vi "Unit Test FGV Spectrometer.vi"() -> ()   [LabVIEW 2013]
doc: "Use this template to build a producer/consumer design pattern with events to produce queue items. Use this design pattern instead of the User Interface Event Handler pattern for user interfaces when you want to execute code asynchronously in response to an event without slowing the user interface responsiveness."
uses:
  FGV Spectro Data.ctl
  Action Spectro.ctl
panel:
  in  "Set Device":bool
  out "Integration Time":dbl
  in  "Get Integration":bool
  in  "Device Set":i32
  out "Data out":T1
  out "Serial Number":string[](array[string])
  in  "Initialize":bool
  in  "Set Integ":dbl
  in  "Set Integration":bool
  in  "Get Spectre":bool
  in  "Disconnect":bool
  in  "Set Averange":bool
  in  "Averange":dbl
  in  "error in (no error)":errorcluster
  in  "Get WaveLength":bool
  out "error out":errorcluster
  in  "Connect":bool
  in  "stop":bool
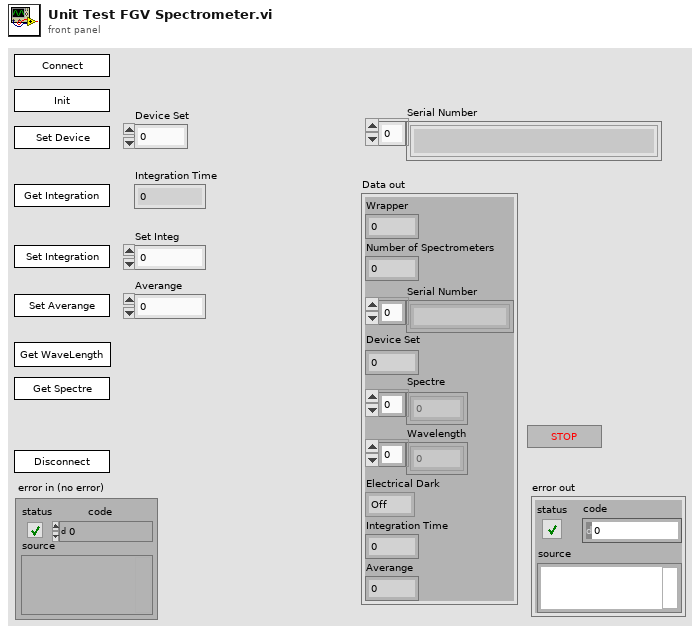
[diagram p1: front panel]
types:
  T1 = typedef "FGV Spectro Data.ctl" = cluster{"Wrapper":u32, "Number of Spectrometers":i32, "Serial Number":string[], "Device Set":i32, "Spectre":dbl[], "Wavelength":dbl[], "Electrical Dark":enum16{"Off", "On"}, "Integration Time":i32, "Averange":i32}
  T2 = typedef "Action Spectro.ctl" = enum16{"Connect", "Initialisation", "Set Device", "Set Intégration time", "Get integration Time", "Disable Noise Suppress", "Enable Noise Suppress", "Set Averange", "Get Spectrum", "Get WaveLength", "Abort", "Disconnect"}
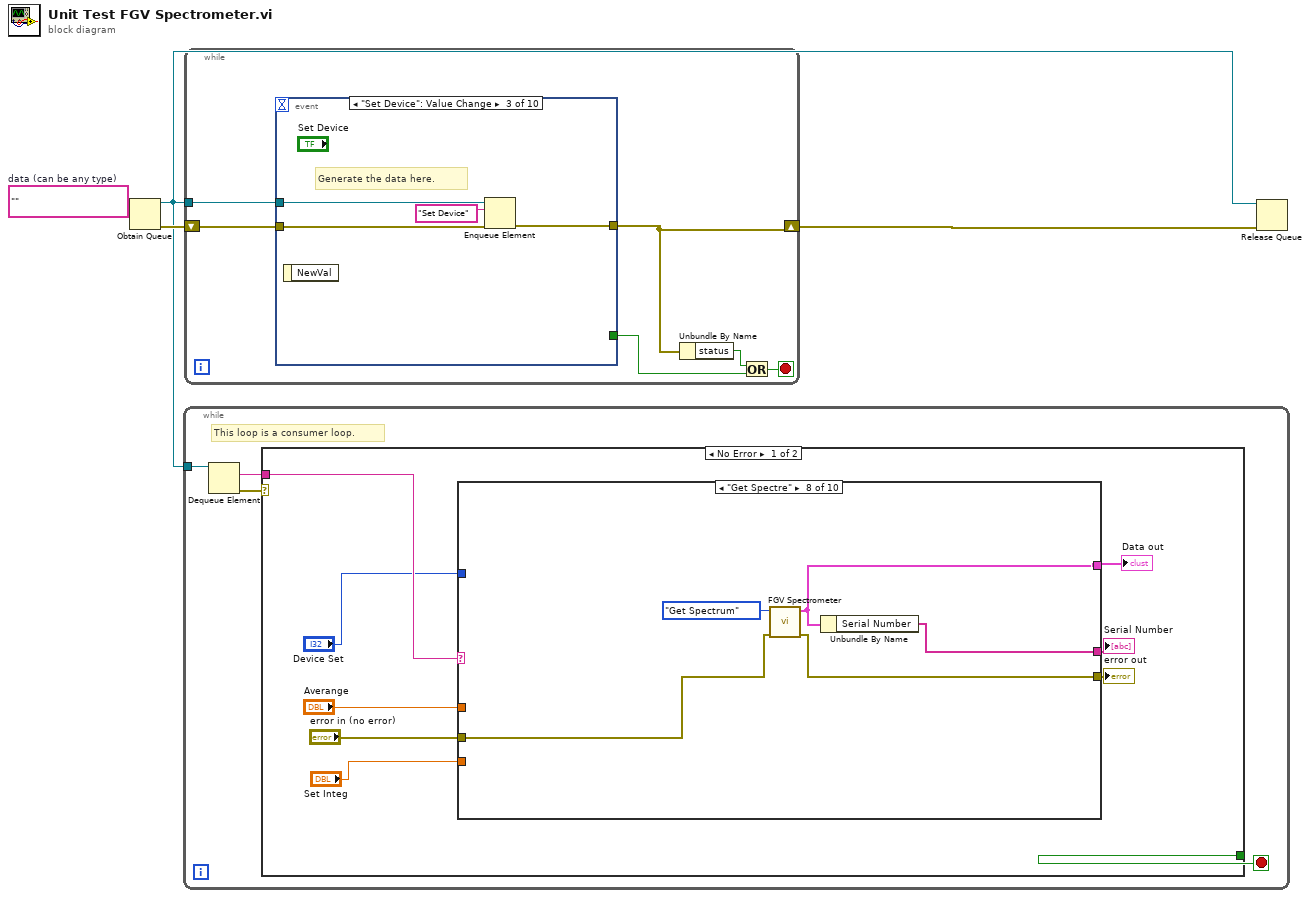
[diagram p0: block diagram]
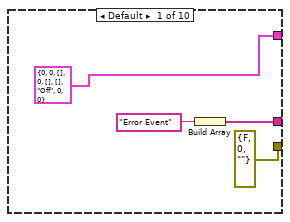
[diagram p2: hidden frame]
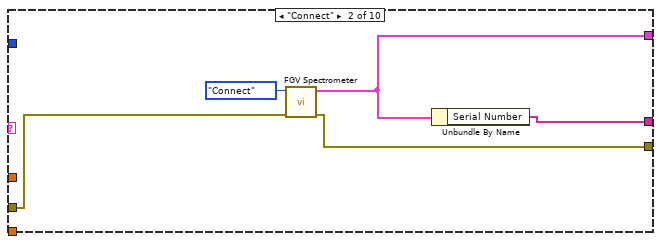
[diagram p3: hidden frame]
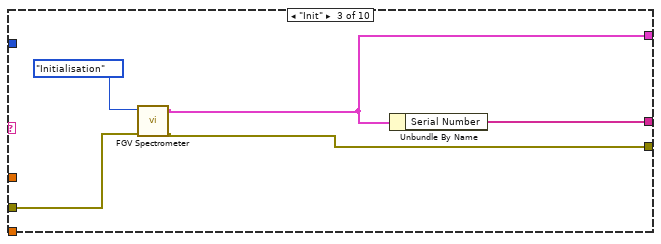
[diagram p4: hidden frame]
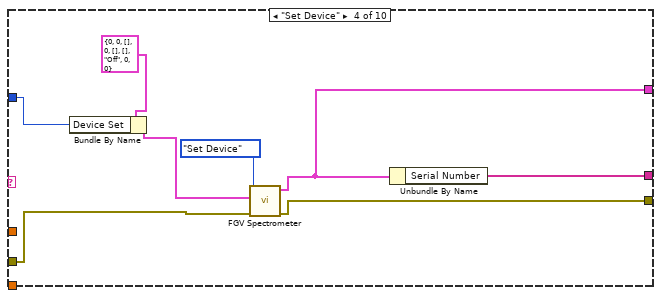
[diagram p5: hidden frame]
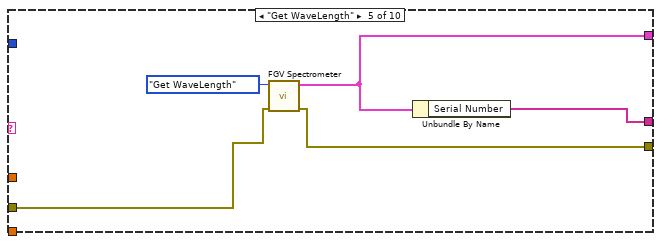
[diagram p6: hidden frame]
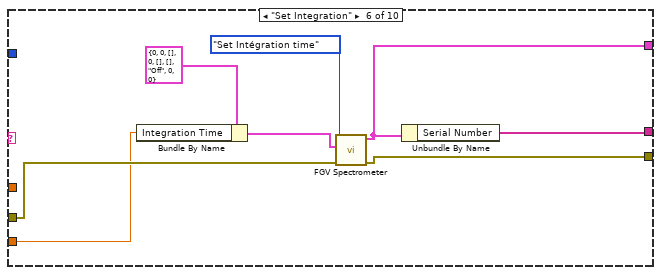
[diagram p7: hidden frame]
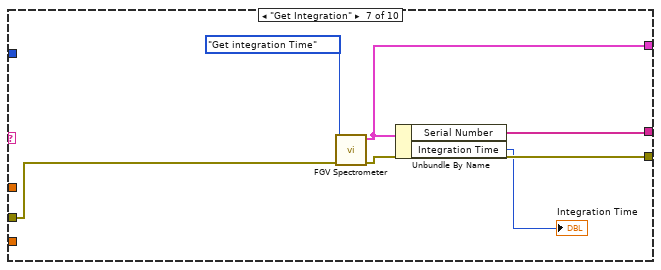
[diagram p8: hidden frame]
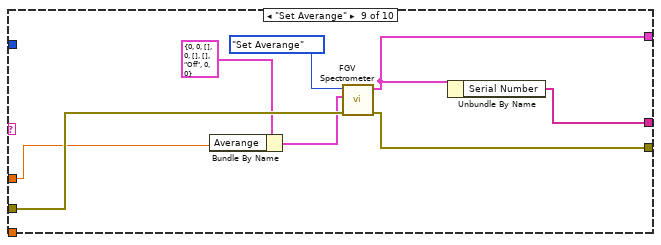
[diagram p9: hidden frame]
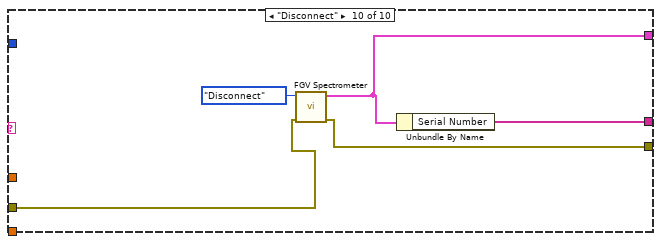
[diagram p10: hidden frame]
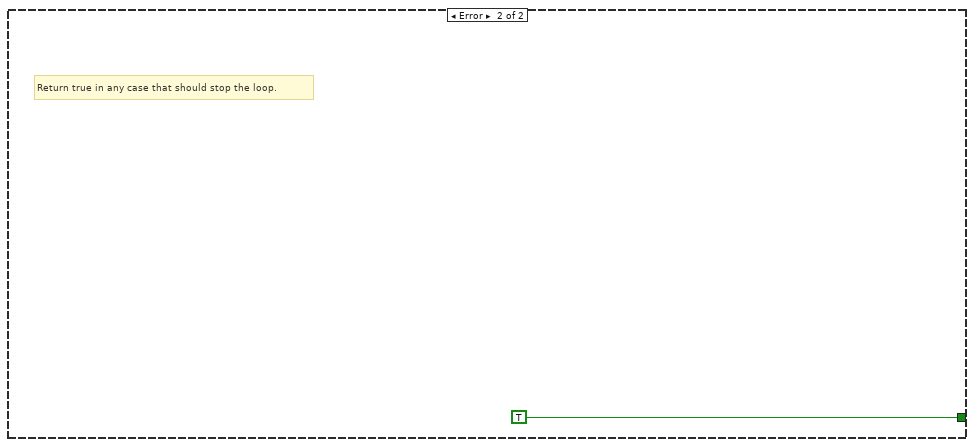
[diagram p11: hidden frame]
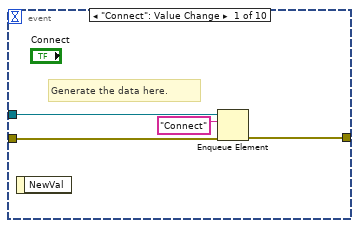
[diagram p12: hidden frame]
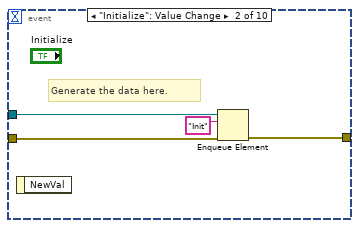
[diagram p13: hidden frame]
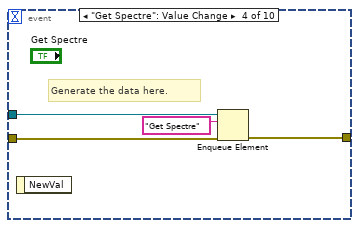
[diagram p14: hidden frame]
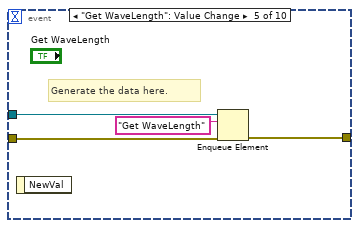
[diagram p15: hidden frame]
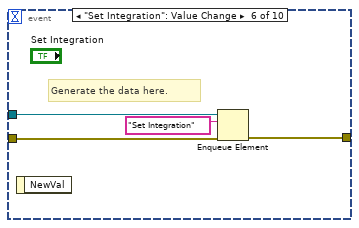
[diagram p16: hidden frame]
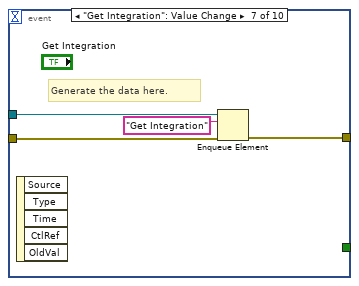
[diagram p17: hidden frame]
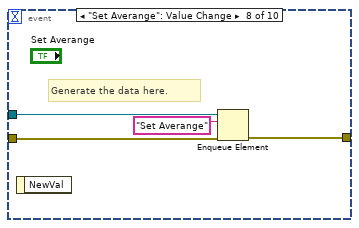
[diagram p18: hidden frame]
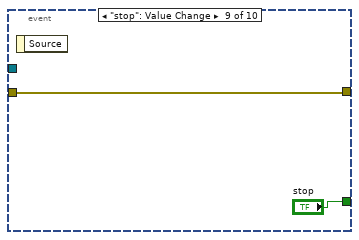
[diagram p19: hidden frame]
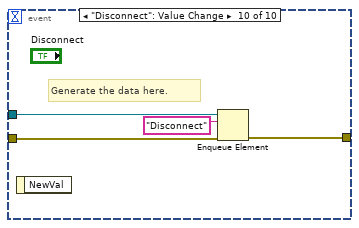
[diagram p20: hidden frame]
diagram:
  w2 = ""  # data (can be any type)
  n1 = Obtain Queue(element data type=w2) -> (queue out=w1:refnum<queue>, error out=w4:errorcluster)  [unwired: 4 in, 1 out]
  n2 = while {
    tunnel: w1 -> [w8]
    stop <- w5 stop-if-true
    # "This loop is a consumer loop."
    n3 = Dequeue Element(queue=w8) -> (element=w6:string, error out=w7:errorcluster)  [unwired: 2 in, 2 out]
    n4 = case shown="No Error" w7 {
      tunnel: w6 -> [w16 _]
      tunnel: [_ TRUE] -> w5
      frame No Error {
        n5 = case shown="\"Get Spectre\"" w16 {
          tunnel: [w17 w24 w29 w31 w41 w50 w56 w59 w67 w73] -> w11
          tunnel: [errorcluster {"status"=FALSE, "code"=0, "source"=""} ("error out") w23 w27 w32 w42 w49 w55 w61 w69 w74] -> w12
          tunnel: "error in (no error)" -> [_ w22 w30 w36 w43 w48 w54 w62 w70 w75]
          tunnel: "Averange" -> [_ _ _ _ _ _ _ _ w64 _]
          tunnel: "Set Integ" -> [_ _ _ _ _ w44 _ _ _ _]
          tunnel: [T1 {"Wrapper"=0, "Number of Spectrometers"=0, "Serial Number"=[], "Device Set"=0, "Spectre"=[], "Wavelength"=[], "Electrical Dark"=enum."Off", "Integration Time"=0, "Averange"=0} ("Data out") w21 w26 w33 w39 w51 w57 w60 w68 w72] -> w10
          tunnel: "Device Set" -> [_ _ _ w35 _ _ _ _ _ _]
          frame Default {
            n6 = Build Array("Error Event" ("Status")) -> (w17:string[])
          }
          frame "Connect" {
            n7 = call "FGV Spectrometer.vi"("entrée d'erreur (pas d'erreur)"=w22, "Action"=Action_Spectro."Connect") -> ("sortie d'erreur"=w23:errorcluster, "Data out"=w21:T1)  [unwired: 8 in]
            n8 = Unbundle By Name(w21) -> ("Serial Number"=w24:string[])
          }
          frame "Init" {
            n9 = call "FGV Spectrometer.vi"("entrée d'erreur (pas d'erreur)"=w30, "Action"=Action_Spectro."Initialisation") -> ("sortie d'erreur"=w27:errorcluster, "Data out"=w26:T1)  [unwired: 8 in]
            n10 = Unbundle By Name(w26) -> ("Serial Number"=w29:string[])
          }
          frame "Set Device" {
            n11 = Bundle By Name(cluster=T1 {"Wrapper"=0, "Number of Spectrometers"=0, "Serial Number"=[], "Device Set"=0, "Spectre"=[], "Wavelength"=[], "Electrical Dark"=enum."Off", "Integration Time"=0, "Averange"=0} ("FGV Spectro. Data"), "Device Set"=w35) -> (w37:T1)
            n12 = call "FGV Spectrometer.vi"("entrée d'erreur (pas d'erreur)"=w36, "FGV Spectro. Data"=w37, "Action"=Action_Spectro."Set Device") -> ("sortie d'erreur"=w32:errorcluster, "Data out"=w33:T1)  [unwired: 7 in]
            n13 = Unbundle By Name(w33) -> ("Serial Number"=w31:string[])
          }
          frame "Get WaveLength" {
            n14 = call "FGV Spectrometer.vi"("entrée d'erreur (pas d'erreur)"=w43, "Action"=Action_Spectro."Get WaveLength") -> ("sortie d'erreur"=w42:errorcluster, "Data out"=w39:T1)  [unwired: 8 in]
            n15 = Unbundle By Name(w39) -> ("Serial Number"=w41:string[])
          }
          frame "Set Integration" {
            n16 = Bundle By Name(cluster=T1 {"Wrapper"=0, "Number of Spectrometers"=0, "Serial Number"=[], "Device Set"=0, "Spectre"=[], "Wavelength"=[], "Electrical Dark"=enum."Off", "Integration Time"=0, "Averange"=0} ("FGV Spectro. Data"), "Integration Time"=w44) -> (w46:T1)
            n17 = call "FGV Spectrometer.vi"("entrée d'erreur (pas d'erreur)"=w48, "FGV Spectro. Data"=w46, "Action"=Action_Spectro."Set Intégration time") -> ("sortie d'erreur"=w49:errorcluster, "Data out"=w51:T1)  [unwired: 7 in]
            n18 = Unbundle By Name(w51) -> ("Serial Number"=w50:string[])
          }
          frame "Get Integration" {
            n19 = call "FGV Spectrometer.vi"("entrée d'erreur (pas d'erreur)"=w54, "Action"=Action_Spectro."Get integration Time") -> ("sortie d'erreur"=w55:errorcluster, "Data out"=w57:T1)  [unwired: 8 in]
            n20 = Unbundle By Name(w57) -> ("Serial Number"=w56:string[], "Integration Time"=→"Integration Time":i32)
          }
          frame "Get Spectre" {
            n21 = call "FGV Spectrometer.vi"("entrée d'erreur (pas d'erreur)"=w62, "Action"=Action_Spectro."Get Spectrum") -> ("sortie d'erreur"=w61:errorcluster, "Data out"=w60:T1)  [unwired: 8 in]
            n22 = Unbundle By Name(w60) -> ("Serial Number"=w59:string[])
          }
          frame "Set Averange" {
            n23 = Bundle By Name(cluster=T1 {"Wrapper"=0, "Number of Spectrometers"=0, "Serial Number"=[], "Device Set"=0, "Spectre"=[], "Wavelength"=[], "Electrical Dark"=enum."Off", "Integration Time"=0, "Averange"=0} ("FGV Spectrometer Data"), "Averange"=w64) -> (w63:T1)
            n24 = call "FGV Spectrometer.vi"("entrée d'erreur (pas d'erreur)"=w70, "FGV Spectro. Data"=w63, "Action"=Action_Spectro."Set Averange") -> ("sortie d'erreur"=w69:errorcluster, "Data out"=w68:T1)  [unwired: 7 in]
            n25 = Unbundle By Name(w68) -> ("Serial Number"=w67:string[])
          }
          frame "Disconnect" {
            n26 = call "FGV Spectrometer.vi"("entrée d'erreur (pas d'erreur)"=w75, "Action"=Action_Spectro."Disconnect") -> ("sortie d'erreur"=w74:errorcluster, "Data out"=w72:T1)  [unwired: 8 in]
            n27 = Unbundle By Name(w72) -> ("Serial Number"=w73:string[])
          }
        }
        "error out" <- w12
        "Serial Number" <- w11
        "Data out" <- w10
      }
      frame Error {
        # "Return true in any case that should stop the loop."
      }
    }
  }
  n28 = while {
    shift-right: [w78] -> w3
    shift-left: w4 -> [w81]
    tunnel: w1 -> [w82]
    stop <- w79 stop-if-true
    n29 = event shown="[2] \"Set Device\": Value Change" {
      selector: _ -> [_ _ _ _ _ _ _ _ _ _]
      dyn-events: _ -> [_ _ _ _ _ _ _ _ _ _]
      timeout: _ -> [_ _ _ _ _ _ _ _ _ _]
      tunnel: w82 -> [w86 w90 w94 w98 w102 w106 w110 w114 _ w120]
      tunnel: w81 -> [w85 w89 w93 w97 w101 w105 w109 w113 w115 w119]
      tunnel: [w84 w88 w92 w96 w100 w104 w108 w112 w115 w118] -> w78
      tunnel: [_ _ _ _ _ _ _ _ "stop" _] -> w80
      event "Connect": Value Change {
        # "Generate the data here."
        n30 = event-data() -> ()  [unwired: 1 in, 1 out]
        n31 = Enqueue Element(queue=w86, element="Connect", error in (no error)=w85) -> (error out=w84:errorcluster)  [unwired: 1 in, 2 out]
      }
      event "Initialize": Value Change {
        # "Generate the data here."
        n32 = event-data() -> ()  [unwired: 1 in, 1 out]
        n33 = Enqueue Element(queue=w90, element="Init", error in (no error)=w89) -> (error out=w88:errorcluster)  [unwired: 1 in, 2 out]
      }
      event "Set Device": Value Change {
        # "Generate the data here."
        n34 = event-data() -> ()  [unwired: 1 in, 1 out]
        n35 = Enqueue Element(queue=w94, element="Set Device", error in (no error)=w93) -> (error out=w92:errorcluster)  [unwired: 1 in, 2 out]
      }
      event "Get Spectre": Value Change {
        # "Generate the data here."
        n36 = event-data() -> ()  [unwired: 1 in, 1 out]
        n37 = Enqueue Element(queue=w98, element="Get Spectre", error in (no error)=w97) -> (error out=w96:errorcluster)  [unwired: 1 in, 2 out]
      }
      event "Get WaveLength": Value Change {
        # "Generate the data here."
        n38 = event-data() -> ()  [unwired: 1 in, 1 out]
        n39 = Enqueue Element(queue=w102, element="Get WaveLength", error in (no error)=w101) -> (error out=w100:errorcluster)  [unwired: 1 in, 2 out]
      }
      event "Set Integration": Value Change {
        # "Generate the data here."
        n40 = event-data() -> ()  [unwired: 1 in, 1 out]
        n41 = Enqueue Element(queue=w106, element="Set Integration", error in (no error)=w105) -> (error out=w104:errorcluster)  [unwired: 1 in, 2 out]
      }
      event "Get Integration": Value Change {
        # "Generate the data here."
        n42 = event-data() -> ()  [unwired: 1 in, 5 out]
        n43 = Enqueue Element(queue=w110, element="Get Integration", error in (no error)=w109) -> (error out=w108:errorcluster)  [unwired: 1 in, 2 out]
      }
      event "Set Averange": Value Change {
        # "Generate the data here."
        n44 = event-data() -> ()  [unwired: 1 in, 1 out]
        n45 = Enqueue Element(queue=w114, element="Set Averange", error in (no error)=w113) -> (error out=w112:errorcluster)  [unwired: 1 in, 2 out]
      }
      event "stop": Value Change {
        n46 = event-data() -> ()  [unwired: 1 in, 1 out]
      }
      event "Disconnect": Value Change {
        # "Generate the data here."
        n47 = event-data() -> ()  [unwired: 1 in, 1 out]
        n48 = Enqueue Element(queue=w120, element="Disconnect", error in (no error)=w119) -> (error out=w118:errorcluster)  [unwired: 1 in, 2 out]
      }
    }
    n49 = Unbundle By Name(w78) -> ("status"=w77:bool)
    n50 = Or(x=w77, y=w80) -> (x .or. y?=w79:bool)
  }
  n51 = Release Queue(queue=w1, error in (no error)=w3) -> ()  [unwired: 1 in, 3 out]
